vi "clearBuffer.vi"(8 "error in (no error)":errorcluster, 11 "Electrometer in":refnum<class "Electrometer.lvclass">) -> (0 "error out":errorcluster, 3 "Electrometer out":refnum<class "Electrometer.lvclass">)   [LabVIEW 2016, in "Electrometer.lvclass"]
uses:
  Electrometer.lvclass
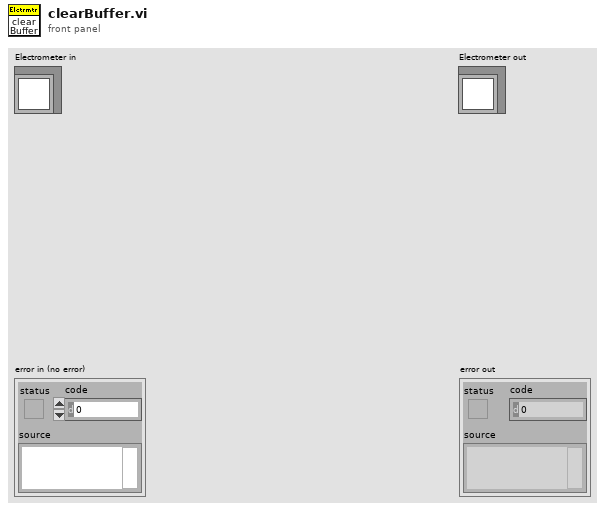
[diagram p1: front panel]
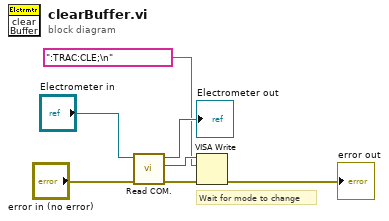
[diagram p0: block diagram]
diagram:
  # "Wait for mode to change"
  n1 = call "Read COM..vi"("error in (no error)"="error in (no error)", "Electrometer in"="Electrometer in") -> ("error out"=w5:errorcluster, "VISA"=w7:refnum<visa-resource-name>, "Electrometer out"=→"Electrometer out":refnum<class "Electrometer.lvclass">)  [unwired: 7 in]
  n2 = VISA Write(VISA resource name=w7, write buffer=":TRAC:CLE;\n", error in (no error)=w5) -> (error out=→"error out":errorcluster)  [unwired: 2 out]
